vi "Turn Turret.vi"(6 "Description":string, 8 "Command Info In":T1, 10 "Turret Angle":dbl, 11 "Synchronication":enum16{"Start", "Wait"}(ring)) -> (0 "Command Info Out":T1)   [LabVIEW 2016]
uses:
  Implementation/Shooter Operations.ctl
  Implementation/Shooter Setpoints.ctl
  <vilib>/Rock Robotics/WPI/Framework/Completion Status.ctl
  <vilib>/Rock Robotics/WPI/Framework/Completion Notifier.ctl
  <vilib>/Rock Robotics/WPI/Framework/Command Status Info.ctl
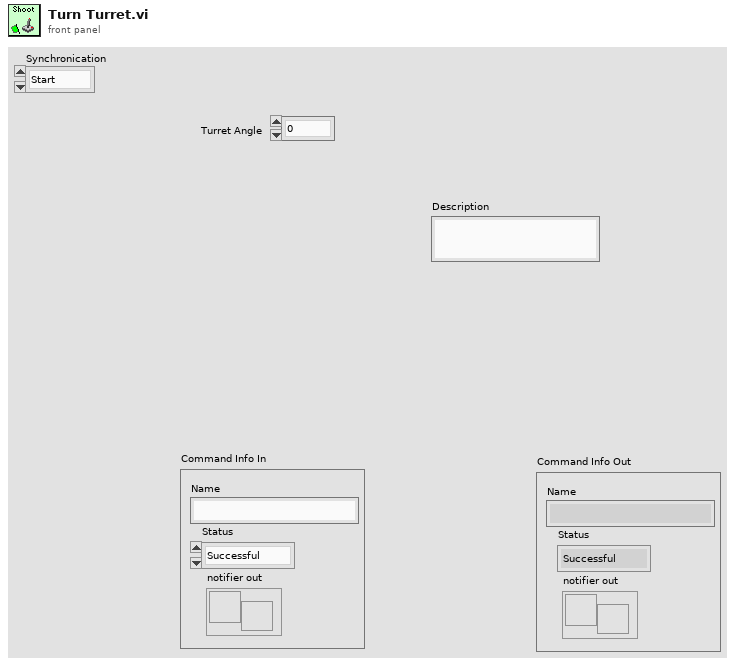
[diagram p1: front panel]
types:
  T1 = typedef "Command Status Info.ctl" = cluster{"Name":string, "Status":T2, "notifier out":T3}
  T2 = typedef "Completion Status.ctl" = enum16{"Successful", "Aborted", "Incomplete"}
  T3 = typedef "Completion Notifier.ctl" = refnum<notifier>
  T4 = typedef "Shooter Operations.ctl" = enum16{"Reserve", "Read Current", "Turn Turret", "Immediate", "Spin Flywheels", "Vision align", "Angle Hood", "Stop flywheels"}
  T5 = typedef "Shooter Setpoints.ctl" = cluster{"Operation":T4, "Setpoint":dbl, "Turret Angle":dbl, "Hood Angle":dbl, "Speed (RPM)":dbl}
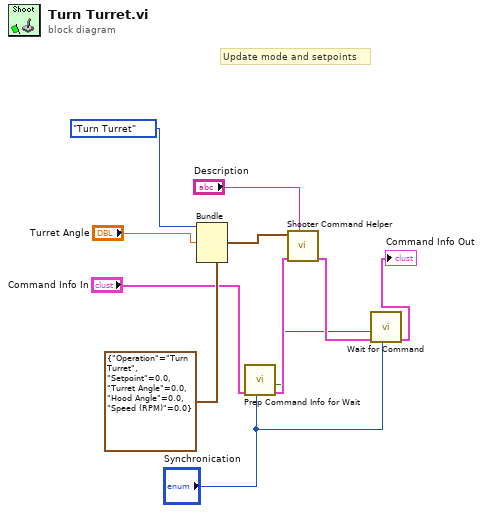
[diagram p0: block diagram]
diagram:
  # "Update mode and setpoints"
  n1 = Bundle(cluster=T5 {"Operation"=enum."Turn Turret", "Setpoint"=0.0, "Turret Angle"=0.0, "Hood Angle"=0.0, "Speed (RPM)"=0.0} ("SubSystem Data"), "Operation"=Shooter_Operations."Turn Turret", "Turret Angle"="Turret Angle") -> (w9:T5)  [unwired: 3 in]
  n2 = call <vilib>:"Prep Command Info for Wait.vi"("Synchronication"="Synchronication", "Command Info"="Command Info In") -> ("Command Info"=w5:T1, "Allocated"=w2:bool)  [unwired: 8 in]
  n3 = call "Shooter Command Helper.vi"("Description"="Description", "Command Info In"=w5, "SubSystem Data"=w9) -> ("Command Info Out"=w4:T1)  [unwired: 7 in, 1 out]
  n4 = call <vilib>:"Wait for Command.vi"("Synchronication"="Synchronication", "Command Info in"=w4, "Allocated"=w2) -> ("Command Info out"=→"Command Info Out":T1)  [unwired: 8 in]
